vi "Close.vi"(8 "error in (no error)":errorcluster, 11 "Thermometer DAQmx Base CFG in":refnum<class "Thermometer DAQmx Base CFG.lvclass">) -> (0 "error out":errorcluster, 3 "Thermometer DAQmx Base CFG out":refnum<class "Thermometer DAQmx Base CFG.lvclass">)   [LabVIEW 2023, in "Thermometer DAQmx Base CFG.lvclass"]
uses:
  Thermometer DAQmx Base CFG.lvclass
  Thermometer DAQmx Base CFG.lvclass/Thermometer DAQmx Base CFG.ctl
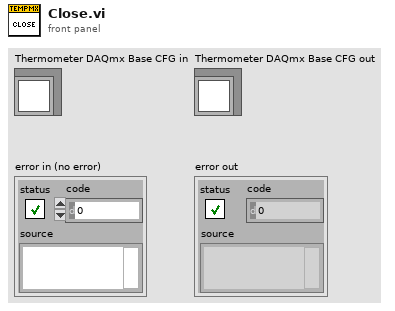
[diagram p1: front panel]
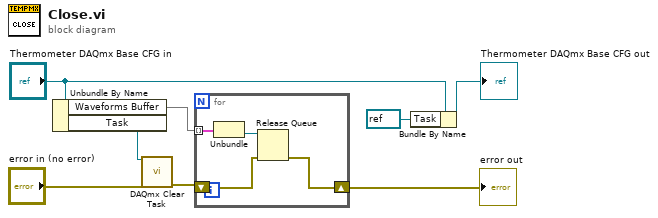
[diagram p0: block diagram]
diagram:
  n1 = Unbundle By Name("Thermometer DAQmx Base CFG in") -> ("Waveforms Buffer"=w3:map{string, refnum<queue>}, "Task"=w7:refnum<k21>)
  n2 = call <vilib>:"DAQmx Clear Task.vi"("task in"=w7, "error in"="error in (no error)") -> ("error out"=w2:errorcluster)  [unwired: 13 in]
  n3 = for {
    tunnel: w3 -> [w12] mode=indexing
    shift-right: [w9] -> w1
    shift-left: w2 -> [w10]
    n4 = Unbundle(w12) -> ("Waveform Queue"=w11:refnum<queue>)  [unwired: 1 out]
    n5 = Release Queue(queue=w11, error in (no error)=w10) -> (error out=w9:errorcluster)  [unwired: 1 in, 2 out]
  }
  "error out" <- w1
  n6 = Bundle By Name(cluster="Thermometer DAQmx Base CFG in", "Task"=refnum<k21> refnum) -> (→"Thermometer DAQmx Base CFG out":refnum<class "Thermometer DAQmx Base CFG.lvclass">)
